vi "FFT ph.vi"(3 "Shift In":cdb[](array[numeric]), 4 "Loop Index":i32, 5 "Array":dbl[](array[numeric])) -> (0 "Shift out":cdb[](array[numeric]), 2 "FFT {X}":cdb[](array[numeric]))   [LabVIEW 2022 SP3]
uses:
  <vilib>/Analysis/2dsp.llb/Real FFT.vi
  <vilib>/Analysis/baseanly.llb/Mean.vi
  <vilib>/Analysis/baseanly.llb/Mean (DBL).vi
  <vilib>/Analysis/NI_AALPro.lvlib
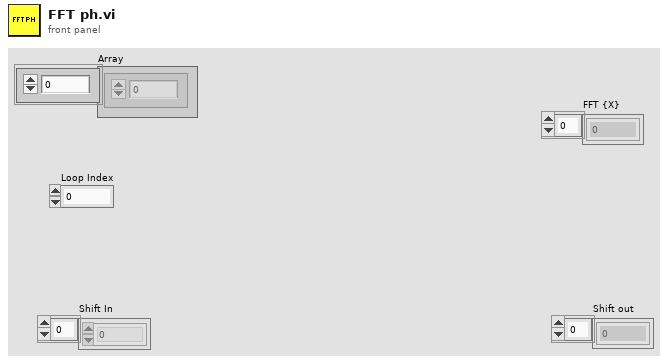
[diagram p1: front panel]
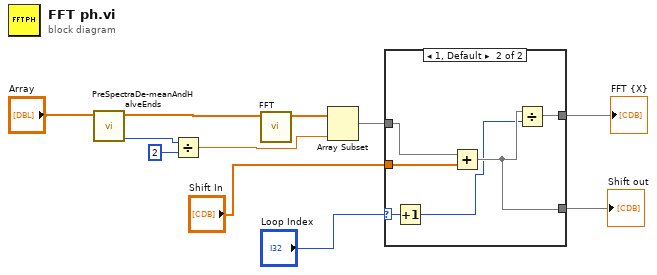
[diagram p0: block diagram]
diagram:
  n1 = call "PreSpectraDe-meanAndHalveEnds.vi"("Array"="Array") -> ("length"=w2:i32, "PreppedArray"=w11:dbl[])  [unwired: 9 in]
  n2 = Divide(x=w2, y=2) -> (x/y=w1:dbl)
  n3 = call-poly <vilib>:"FFT.vi"("X"=w11) -> ("FFT {X}"=w9:cdb[])  [unwired: 9 in, 1 out]
  n4 = Array Subset(array=w9, length=w1) -> (w6:cdb[])  [unwired: 1 in]
  n5 = case shown="1, Default" "Loop Index" {
    selector: "Loop Index" -> [_ w14]
    tunnel: [w12 w16] -> w7
    tunnel: w6 -> [w12 w18]
    tunnel: [w12 w15] -> w5
    tunnel: "Shift In" -> [_ w17]
    frame 0 {
    }
    frame 1, Default {
      n6 = Increment(x=w14) -> (x+1=w13:i32)
      n7 = Add(x=w18, y=w17) -> (x+y=w16:cdb[])
      n8 = Divide(x=w16, y=w13) -> (x/y=w15:cdb[])
    }
  }
  "Shift out" <- w7
  "FFT {X}" <- w5
